vi "Housekeeping Management.vi"(11 "CIFPluginManager in":refnum<class "CIFPluginManager.lvclass">) -> (0 "error out":errorcluster)   [LabVIEW 2021, in "CIFPluginManager.lvclass"]
uses:
  CIFPluginManager.lvclass
  CIFPluginManager.lvclass/CIFPluginManager.ctl
  CIFUtilities/CIFLogs/CIFLogs.lvlib
  gRPC/CIF_Manager_Client_Wrapper/CIFManagerClientWrapper.lvlib
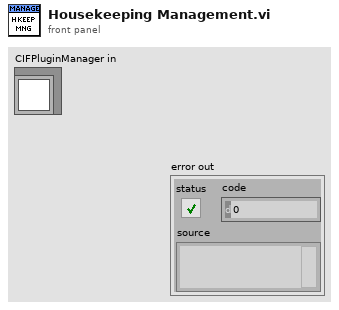
[diagram p1: front panel]
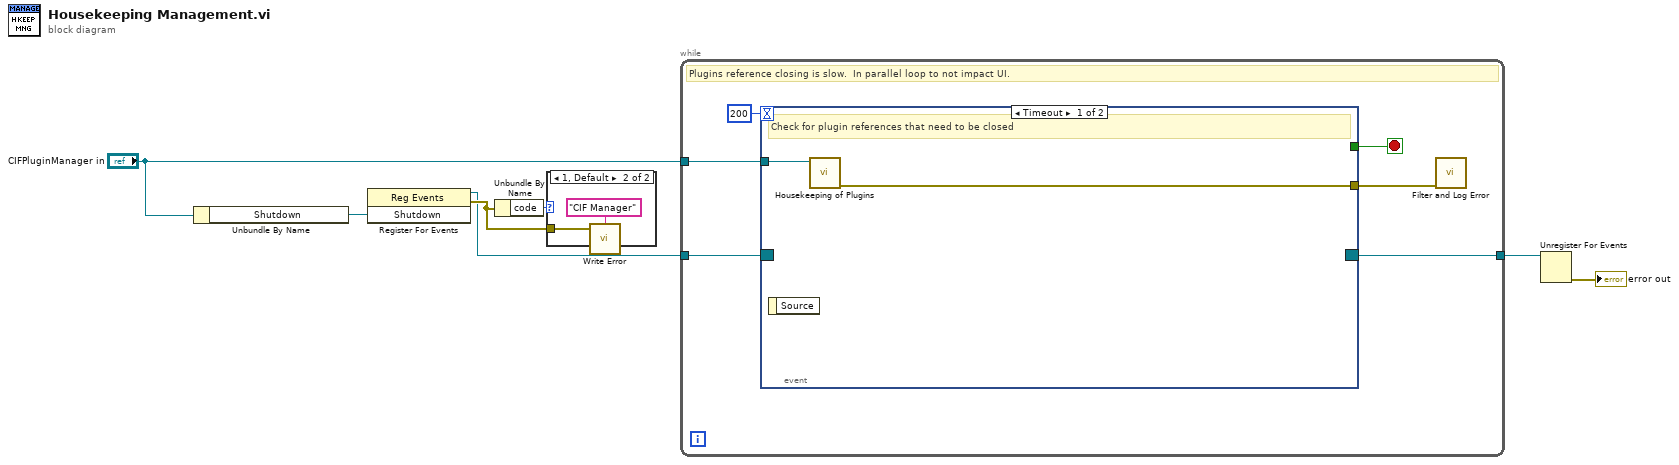
[diagram p0: block diagram]
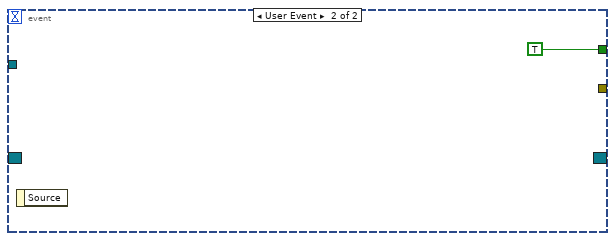
[diagram p3: hidden frame]
diagram:
  n1 = Unbundle By Name("CIFPluginManager in") -> ("Shutdown"=w2:refnum<user-event>)
  n2 = register-events(w2) -> (reference out=w3:refnum<event-registration>, error out=w4:errorcluster)  [unwired: 2 in]
  n3 = Unbundle By Name(w4) -> ("code"=w5:i32)
  n4 = case shown="1, Default" w5 {
    tunnel: w4 -> [_ w9]
    frame 0 {
      # "-1001 is cancelled by client.  Not an error."
    }
    frame 1, Default {
      n5 = call "Write Error.vi"("error in (no error)"=w9, "Plugin Name"="CIF Manager") -> ()  [unwired: 2 in, 1 out]
    }
  }
  n6 = while {
    tunnel: w3 -> [w10]
    tunnel: [w12] -> w6
    tunnel: "CIFPluginManager in" -> [w15]
    stop <- w13 stop-if-true
    # "Plugins reference closing is slow.  In parallel loop to not impact UI."
    n7 = event shown="[0] Timeout" {
      selector: w10 -> [_ _]
      dyn-events: [_ _] -> w12
      timeout: 200 -> [_ _]
      tunnel: w15 -> [w16 _]
      tunnel: [_ TRUE] -> w13
      tunnel: [w17 _] -> w11
      event Timeout {
        # "Check for plugin references that need to be closed"
        n8 = event-data() -> ()  [unwired: 1 in, 1 out]
        n9 = call "Housekeeping of Plugins.vi"("CIFPluginManager in"=w16) -> ("error out"=w17:errorcluster)  [unwired: 10 in]
      }
      event User Event {
        n10 = event-data() -> ()  [unwired: 1 in, 1 out]
      }
    }
    n11 = call "Filter and Log Error.vi"("error In"=w11) -> ()  [unwired: 11 in]
  }
  n12 = Unregister For Events(event registration refnum=w6) -> (error out=→"error out":errorcluster)  [unwired: 1 in]
